vi "Valid Path__ogtk.vi"   [LabVIEW 2009]
doc: "This polymorphic VI checks whether path (or array of paths) is valid, meaning not \"Empty path\" and not \"Not a Path\"."
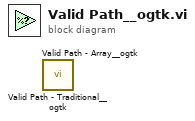
[diagram p0: block diagram]
diagram:
  n1 = call "Valid Path - Traditional__ogtk.vi"() -> ()  [unwired: 1 in, 1 out]
  n2 = call "Valid Path - Array__ogtk.vi"() -> ()  [unwired: 1 in, 1 out]
